vi "get_settings_paths.vi"(8 "error in (no error)":errorcluster, 10 "file name":string, 11 "GenericComponent in":refnum<class "GenericComponent.lvclass">) -> (0 "error out":errorcluster, 1 "settings file path":path, 2 "settings folder for a specific component":path, 3 "GenericComponent out":refnum<class "GenericComponent.lvclass">, 5 "settings base folder for a specific user":path, 7 "settings base folder":path)   [LabVIEW 2017, in "GenericComponent.lvclass"]
uses:
  GenericComponent.lvclass
  xcontrols/XUserDropdown/XUserDropdown/XUserDropdown.xctl
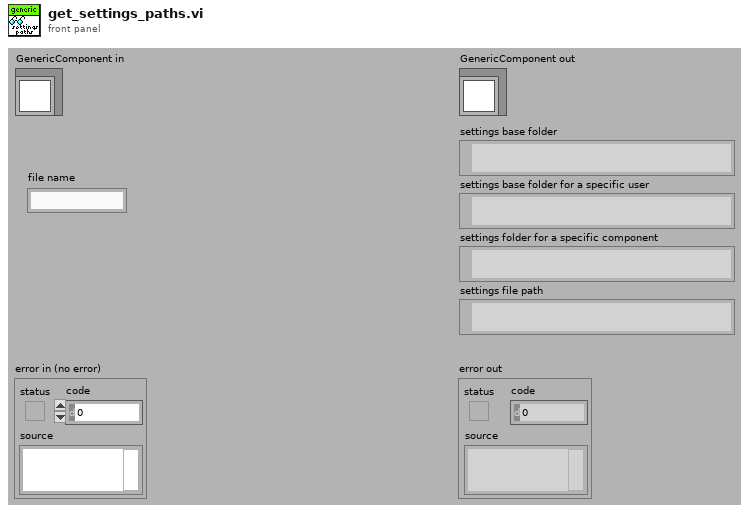
[diagram p1: front panel]
types:
  T1 = typedef "plugin_specification.ctl" = cluster{"class path":string, "configuration":string, "label":string, "settings name":string}
  T2 = typedef "settings_paths_cluster.ctl" = cluster{"base folder":path, "base folder for user":path, "component folder":path, "component file path":path}
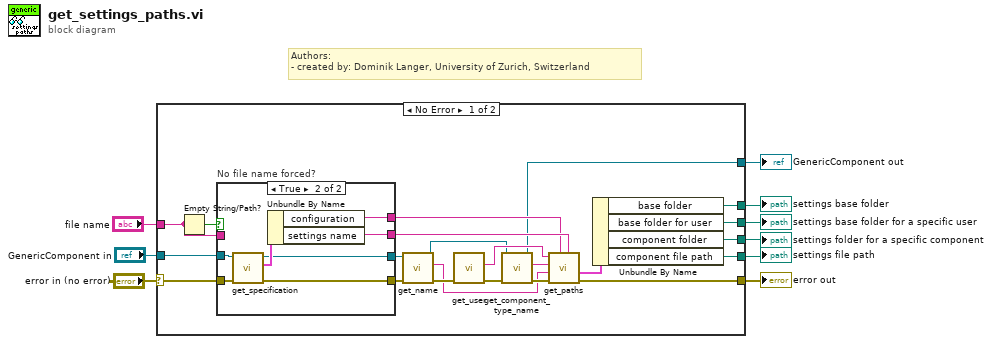
[diagram p0: block diagram]
diagram:
  # "Authors: \n- created by: Dominik Langer, University of Zurich, Switzerland"
  n1 = case shown="No Error" "error in (no error)" {
    selector: "error in (no error)" -> [w20 w43]
    tunnel: [w19 w43] -> w8
    tunnel: [w12 w42] -> w6
    tunnel: "GenericComponent in" -> [w13 w42]
    tunnel: [w17 _] -> w5
    tunnel: [w16 _] -> w4
    tunnel: [w15 _] -> w3
    tunnel: [w14 _] -> w2
    tunnel: "file name" -> [w11 _]
    frame No Error {
      n2 = Empty String/Path?(string/path=w11) -> (empty?=w31:bool)
      n3 = case "No file name forced?" shown="True" w31 {
        tunnel: w20 -> [w33 w41]
        tunnel: [w33 w39] -> w23
        tunnel: w13 -> [w34 w40]
        tunnel: [w32 w36] -> w21
        tunnel: [w34 w35] -> w24
        tunnel: w11 -> [w32 _]
        tunnel: [w32 w37] -> w22
        frame False {
        }
        frame True {
          n4 = call-dynamic "get_specification.vi"("error in (no error)"=w41, "GenericPlugin in"=w40) -> ("error out"=w39:errorcluster, "component specification"=w38:T1, "GenericPlugin out"=w35:refnum<class "GenericComponent.lvclass">)  [unwired: 6 in, 1 out]
          n5 = Unbundle By Name(w38) -> ("configuration"=w36:string, "settings name"=w37:string)
        }
      }
      n6 = call-dynamic "get_name.vi"("error in (no error)"=w23, "GenericPlugin in"=w24) -> ("error out"=w26:errorcluster, "component name"=w25:string, "GenericPlugin out"=w10:refnum<class "GenericComponent.lvclass">)  [unwired: 7 in]
      n7 = call "get_user.vi"("error in (no error)"=w26) -> ("error out"=w27:errorcluster, "username out"=w28:string)  [unwired: 9 in]
      n8 = call-dynamic "get_component_type_name.vi"("error in (no error)"=w27, "GenericPlugin in"=w10) -> ("error out"=w30:errorcluster, "component type"=w29:string, "GenericPlugin out"=w12:refnum<class "GenericComponent.lvclass">)  [unwired: 7 in]
      n9 = call "get_paths.vi"("settings file name (without ending)"=w22, "configuration file name (without ending)"=w21, "error in (no error)"=w30, "component name"=w25, "component type"=w29, "user"=w28) -> ("error out"=w19:errorcluster, "settings paths"=w18:T2)  [unwired: 2 in, 2 out]
      n10 = Unbundle By Name(w18) -> ("base folder"=w17:path, "base folder for user"=w16:path, "component folder"=w15:path, "component file path"=w14:path)
    }
    frame Error {
    }
  }
  "error out" <- w8
  "GenericComponent out" <- w6
  "settings base folder" <- w5
  "settings base folder for a specific user" <- w4
  "settings folder for a specific component" <- w3
  "settings file path" <- w2
